vi "tx2203.vi"() -> ()   [LabVIEW 2014]
uses:
  <instrlib>/niUSRP/niUSRP Write Tx Data (CDB).vi
panel:
  in  "timeout":dbl=10.0
  out "IQ Plot":dbl[](graph)
  in  "device name":refnum<k15>="192.168.10.2"
  out "Error Out":errorcluster
  in  "active antenna":string="TX/RX"
  in  "Stop Button":bool
  out "Waveform Graph":dbl[](graph)
  out "Gain [dB] (actual)":dbl format="%#.6p"
  out "Carrier Frequency \n[Hz] (actual)":dbl=2450000000.0 format="%#.6p"
  out "IQ Sampling\nRate [s/sec] (actual)":dbl=10000000.0 format="%#.6p"
  in  "Gain [dB]":dbl format="%#.6p"
  in  "Carrier\nFrequency [Hz]":dbl=915000000.0 format="%#.6p"
  in  "IQ Sampling\nRate [s/sec]":dbl=10000000.0 format="%#.6p"
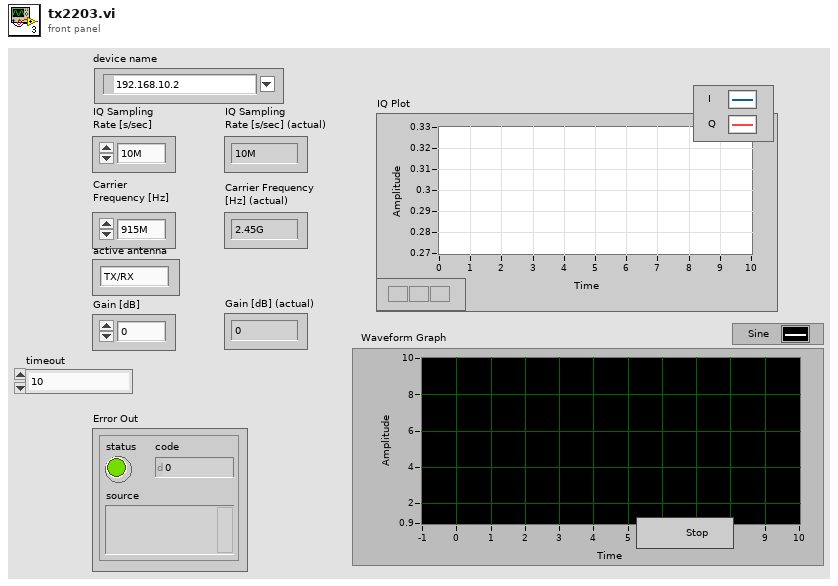
[diagram p1: front panel]
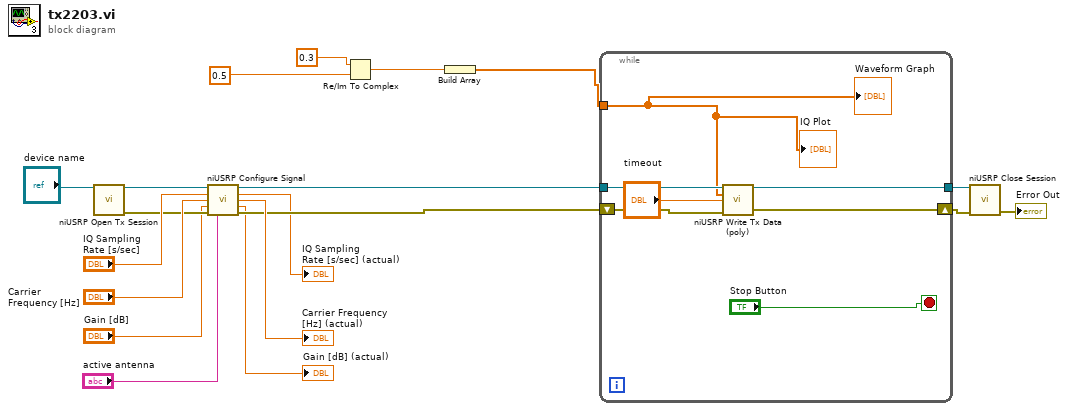
[diagram p0: block diagram]
diagram:
  n1 = call <instrlib>:"niUSRP Open Tx Session.vi"("device names"="device name") -> ("session handle out"=w19:refnum<k15>, "error out"=w16:errorcluster)  [unwired: 13 in]
  n2 = call <instrlib>:"niUSRP Configure Signal.vi"("session handle"=w19, "IQ rate"="IQ Sampling\nRate [s/sec]", "carrier frequency"="Carrier\nFrequency [Hz]", "gain"="Gain [dB]", "error in (no error)"=w16, "active antenna"="active antenna") -> ("session handle out"=w14:refnum<k15>, "coerced IQ rate"=→"IQ Sampling\nRate [s/sec] (actual)":dbl, "coerced carrier frequency"=→"Carrier Frequency \n[Hz] (actual)":dbl, "coerced gain"=→"Gain [dB] (actual)":dbl, "error out"=w13:errorcluster)  [unwired: 5 in]
  n3 = Re/Im To Complex(1:0.5, 2:0.3) -> (0:w5:cdb)
  n4 = Build Array(w5) -> (w4:cdb[])
  n5 = while {
    tunnel: w14 -> [w26]
    tunnel: [w24] -> w12
    tunnel: w4 -> [w22]
    shift-right: [w21] -> w1
    shift-left: w13 -> [w25]
    stop <- "Stop Button" stop-if-true
    n6 = call-poly <instrlib>:"niUSRP Write Tx Data (poly).vi"("session handle"=w26, "data"=w22, "timeout"="timeout", "error in (no error)"=w25) -> ("session handle out"=w24:refnum<k15>, "error out"=w21:errorcluster)  [unwired: 10 in]
    "Waveform Graph" <- w22
    "IQ Plot" <- w22
  }
  n7 = call <instrlib>:"niUSRP Close Session.vi"("session handle"=w12, "error in (no error)"=w1) -> ("error out"=→"Error Out":errorcluster)  [unwired: 13 in]
